vi "Get SMO HELP.vi"(8 "error in (no error)":errorcluster, 10 "Command":string, 11 "Inst.TC in":refnum<class "Inst.TC.lvclass">) -> (0 "error out":errorcluster, 2 "help cluster":T1, 3 "Inst.TC out":refnum<class "Inst.TC.lvclass">)   [LabVIEW 2019, in "Inst.TC.lvclass"]
uses:
  Inst.TC.lvclass
  <userlib>/LevyLab/Instrument Framework/subsystems/Help/typedefs/Help--cluster.ctl
  <userlib>/LevyLab/Instrument Framework/Instrument Types/Cryostat/Instrument.Cryostat.lvclass
  <userlib>/LevyLab/Instrument Framework/subsystems/Help/Help.lvclass
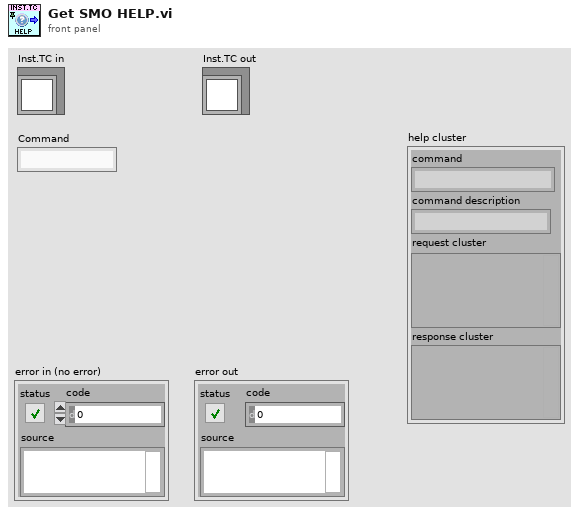
[diagram p1: front panel]
types:
  T1 = typedef "Instrument.lvlib/Help.lvclass/Help--cluster.ctl" = cluster{"command":string, "command description":string, "request cluster":variant, "response cluster":variant}
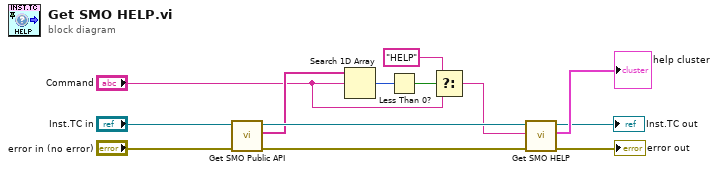
[diagram p0: block diagram]
diagram:
  n1 = call-dynamic "Get SMO Public API.vi"("error in (no error)"="error in (no error)", "Inst.TC in"="Inst.TC in") -> ("error out"=w7:errorcluster, "Commands"=w6:string[], "Inst.TC out"=w9:refnum<class "Inst.TC.lvclass">)  [unwired: 7 in]
  n2 = Search 1D Array(1D array=w6, element="Command") -> (index of element=w5:i32)  [unwired: 1 in]
  n3 = Less Than 0?(x=w5) -> (x < 0?=w4:bool)
  n4 = Select(t="HELP", s=w4, f="Command") -> (s? t:f=w2:string)
  n5 = call-parent "Get SMO HELP.vi"("error in (no error)"=w7, "Command"=w2, "Instrument.Cryostat in"=w9) -> ("error out"=→"error out":errorcluster, "help cluster"=→"help cluster":T1, "Instrument.Cryostat out"=→"Inst.TC out":refnum<class "Inst.TC.lvclass">)  [unwired: 6 in]
